vi "Async Math Example.vi"() -> ()   [LabVIEW 2020, in "Futures-Examples.lvlib"]
uses:
  Futures-Examples.lvlib
  StringValue/StringValue.lvclass
  Promises/Future/Future.lvclass
  DoubleValue/DoubleValue.lvclass
  Promises/Promise/Promise.lvclass
panel:
  in  "Timeout mS":i32=2100
  out "Value":string
  in  "Cause Fail":bool
  out "Resolved Error":errorcluster
  # "Expected operation:\n12 * (7 + 5) + 5\n= 149"
  # "Each task has a 400-600mS wait in it, plus resolving time. So a timeout of 2000mS or less will error but 1902+mS will succeed on a decent computer but 1900mS will timeout."
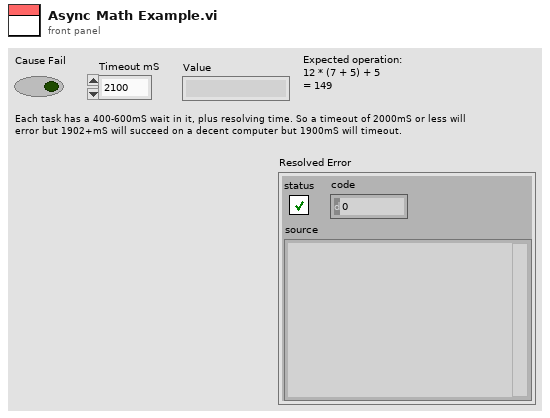
[diagram p1: front panel]
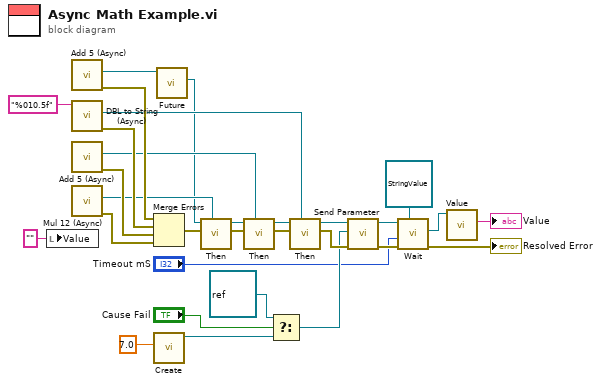
[diagram p0: block diagram]
diagram:
  n1 = local write "Value"("" ("Value")) -> ()
  n2 = call "Add 5 (Async).vi"() -> ("error out"=w28:errorcluster, "Add 5 Promise"=w24:refnum<class "Promise.lvclass">)  [unwired: 10 in]
  n3 = call "DBL to String (Async).vi"("Format String"="%010.5f") -> ("error out"=w27:errorcluster, "Promise out"=w5:refnum<class "Promise.lvclass">)  [unwired: 9 in]
  n4 = call "Add 5 (Async).vi"() -> ("error out"=w26:errorcluster, "Add 5 Promise"=w21:refnum<class "Promise.lvclass">)  [unwired: 10 in]
  n5 = call "Mul 12 (Async).vi"() -> ("error out"=w25:errorcluster, "Mul 12 Promise"=w23:refnum<class "Promise.lvclass">)  [unwired: 10 in]
  n6 = Merge Errors(w28, w27, w26, w25) -> (w16:errorcluster)
  n7 = call "Create.vi"("Value"=7.0) -> ("DoubleValue"=w19:refnum<class "DoubleValue.lvclass">)  [unwired: 10 in]
  n8 = call "Future.vi"("Promise in"=w24) -> ("Future"=w4:refnum<class "Future.lvclass">)  [unwired: 9 in, 1 out]
  n9 = call "Then.vi"("Then Promise"=w23, "error in (no error)"=w16, "Future in"=w4) -> ("error out"=w17:errorcluster, "Future out"=w22:refnum<class "Future.lvclass">)  [unwired: 7 in]
  n10 = call "Then.vi"("Then Promise"=w21, "error in (no error)"=w17, "Future in"=w22) -> ("error out"=w12:errorcluster, "Future out"=w13:refnum<class "Future.lvclass">)  [unwired: 7 in]
  n11 = Select(t=refnum<class> refnum ("LabVIEW Object"), s="Cause Fail", f=w19) -> (s? t:f=w15:refnum<class>)
  n12 = call "Then.vi"("Then Promise"=w5, "error in (no error)"=w12, "Future in"=w13) -> ("error out"=w29:errorcluster, "Future out"=w3:refnum<class "Future.lvclass">)  [unwired: 7 in]
  n13 = call "Send Parameter.vi"("error in (no error)"=w29, "Value"=w15, "Future in"=w3) -> ("error out"=w30:errorcluster, "Future in"=w2:refnum<class "Future.lvclass">)  [unwired: 7 in]
  n14 = call "Wait.vi"("Result Type (None)"=refnum<class "StringValue.lvclass"> refnum ("Futures-Examples.lvlib:StringValue.lvclass"), "error in (no error)"=w30, "Timeout mS (-1)"="Timeout mS", "Future in"=w2) -> ("error out"=→"Resolved Error":errorcluster, "Result"=w10:refnum<class "StringValue.lvclass">)  [unwired: 6 in]
  n15 = call "Value.vi"("StringValue in"=w10) -> ("Value"=→"Value":string)  [unwired: 10 in]
